vi "ABR3-Init Freq.vi"(0 "StimChans":T5[](xcontrol), 1 "Runtime":T28={"Ceiling"=0.0, "Threshold"=0.0, "Crossed?"=FALSE, "Step"=0, "Stop"=0, "Avgs"=0, "Level"=0.0, "AI Npts"=0, "Doubled?"=FALSE, "Gain"=0.0, "NWindowPts"=0, "dt"=0.0, "Cal"=path "", "Freq"=0.0, "AO Channels"=[], "AltPol"=FALSE, "AO Npts"=0, "AO Fs"=0.0, "Start"=0, "Stop max"=0, "Ear"=enum."Right", "Waveform"=enum."TONE PIP", "RepRate"=0.0, "CAP or ABR"=1, "LMasker"=0.0, "SeqVar"=enum."Signal Level", "Reps/buffer"=0, "Avg Mode"=enum."Neural/CM", "Wav"=path "", "Order"=enum."Sequential", "Levels"=[], "ControlVal"=0.0, "innerIndex"=0, "indexStep"=0} {"CAP or ABR" items=["CAP", "ABR"]}, 2 "State (in)":T2, 7 "outerVal":cluster{"wavfile":path, "freq":dbl}, 11 "error in (no error)":errorcluster, 12 "Response":T32={"Gain"=10000, "Averages"=1, "Window (ms)"=512.0, "Thr Fast Steps"=8.5, "AI Fs"=0.0} {"Thr Fast Steps" format="%.2f"; "Window (ms)" format="%.2f"}, 13 "Controls":T1) -> (3 "Runtime out":T28={"Ceiling"=0.0, "Threshold"=0.0, "Crossed?"=FALSE, "Step"=0, "Stop"=0, "Avgs"=0, "Level"=0.0, "AI Npts"=0, "Doubled?"=FALSE, "Gain"=0.0, "NWindowPts"=0, "dt"=0.0, "Cal"=path "", "Freq"=0.0, "AO Channels"=[], "AltPol"=FALSE, "AO Npts"=0, "AO Fs"=0.0, "Start"=0, "Stop max"=0, "Ear"=enum."Right", "Waveform"=enum."TONE PIP", "RepRate"=0.0, "CAP or ABR"=1, "LMasker"=0.0, "SeqVar"=enum."Signal Level", "Reps/buffer"=0, "Avg Mode"=enum."Neural/CM", "Wav"=path "", "Order"=enum."Sequential", "Levels"=[], "ControlVal"=0.0, "innerIndex"=0, "indexStep"=0} {"CAP or ABR" items=["CAP", "ABR"]}, 4 "Stimulus (out)":T5[](xcontrol), 8 "Masker Level":T3, 10 "Ceiling":dbl, 15 "error out":errorcluster)   [LabVIEW 2020]
uses:
  TypeDefs/ABR3-Response.ctl
  epl-vi-lib/Signal Synthesis VIs/Controls/Multichannel (Full)/Multichannel (Full).xctl
  TypeDefs/ABR3-Runtime Data.ctl
  epl-vi-lib/Utility VIs/Type Defs/Left-Right ring.ctl
  TypeDefs/ABR-Waveform Enum.ctl
  TypeDefs/ABR3-Seq Var Enum.ctl
  epl-vi-lib/Signal Synthesis VIs/Controls/Level XCtl/Level Data.ctl
  epl-vi-lib/Signal Synthesis VIs/Controls/Level XCtl/Level Units.ctl
  CFTS Main Panel SubVIs/CFTS-Experiment State.ctl
  TypeDefs/ABR3-Controls.ctl
  epl-vi-lib/Signal Synthesis VIs/Controls/Waveform XCtl/Waveform Enum.ctl
  epl-vi-lib/Signal Synthesis VIs/Top Level VIs/Stimulus-Initialize (full).vi
  epl-vi-lib/Signal Synthesis VIs/Controls/Level XCtl/Level XCtl.xctl
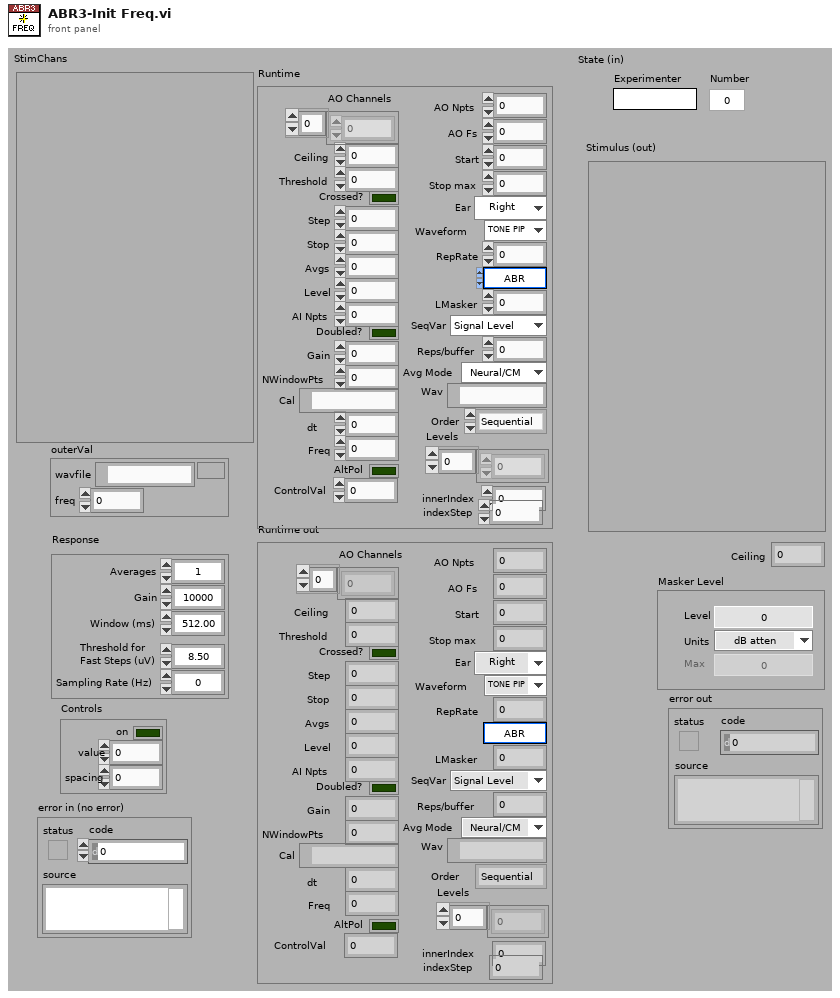
[diagram p1: front panel]
types:
  T1 = typedef "ABR3-Controls.ctl" = cluster{"on":bool, "value":dbl, "spacing":i32}
  T2 = typedef "CFTS-Experiment State.ctl" = cluster{"Experimenter":string, "Number":u32, "Right":string, "Left":string, "Data Folder":path, "State File":path, "Version Info":string, "End Exposure Time":dbl, "Exposure Duration":string, "Run #":cluster{"CAP":i16, "ABR":i16, "DP":i16, "VsEP":i16, "MeasSeq":i16, "SubSeq":i16, "SFOAE":i16}}
  T3 = typedef "Level XCtl.xctl/Level Data.ctl" = cluster{"Level":dbl, "Units":T4, "Max":dbl, "Multiplier":dbl, "Cal File":path, "Cal":cluster{"Freq (Hz)":dbl[], "Mag (dB SPL)":dbl[], "Phase (deg)":dbl[]}}
  T4 = typedef "Level Units.ctl" = enum16{"dB atten", "dB SPL", "dB re 1 Vrms", "dB V/Hz½", "mW", "dB HL", "Volts", "dB mW"}
  T5 = typedef "Stimulus Channel (Full).xctl/Full Stimulus Channel Data.ctl" = cluster{"Waveform":T6, "Filter":T23, "Burst":T25, "Level":T3, "Name":string, "Advanced":T26, "SAM":T27}
  T6 = typedef "Waveform XCtl.xctl/Waveform Data.ctl" = cluster{"Type":T7, "Tone":T8, "Pulse Train":T9, "Noise":T12, "File":T13, "FMSweep":T14, "Chirp Train":T15, "Complex Tone":cluster{"Params":T17, "Data":T19}, "Moving Ripple":T20}
  T7 = typedef "Waveform Enum.ctl" = enum16{"OFF", "Tone", "Noise", "Pulse Train", "File", "FM Sweep", "Chirp Train", "Complex Tone", "FM Tone", "Moving Ripple"}
  T8 = typedef "Tone Params.ctl" = cluster{"Frequency (kHz)":dbl, "Last Freq":dbl, "Last Phase":dbl}
  T9 = typedef "Pulse Train Params.ctl" = cluster{"Pulse width (us)":dbl, "Pulse rate (Hz)":dbl, "Gap (ms)":dbl, "Polarity":T10, "PT State":T11, "Asynch":bool}
  T10 = typedef "Pulse Polarity.ctl" = enum16{"POS", "NEG", "POS-NEG", "NEG-POS"}
  T11 = typedef "PT-Continuous State.ctl" = cluster{"Template":dbl[], "Nperiod":i32, "Index":i32, "Pulse Rate (Hz)":dbl, "Phase (cycles)":dbl, "Noff":i32}
  T12 = typedef "Noise Params.ctl" = cluster{"InvFilt":bool, "Noise":dbl[], "CurPt":i32, "Aweight":bool, "Seed":i32, "afile":path}
  T13 = typedef "StimFile-Params.ctl" = cluster{"Filename":path, "Signal":dbl[], "Channel":i32, "stream":bool, "offset":i32, "nreps":i32, "loops":i32, "Randomize":bool, "order":i32[], "Seed":i32, "Tokens":i32}
  T14 = typedef "FM Sweep Params.ctl" = cluster{"Rate (oct/s)":dbl, "Fmin (Hz)":dbl, "Fmax (Hz)":dbl, "Ramp (ms)":dbl, "Linear":bool}
  T15 = typedef "Chirp Train.ctl" = cluster{"Params":T16, "Data":cluster{"WF":dbl[]}}
  T16 = typedef "Chirp Train Params.ctl" = cluster{"Fmin (kHz)":dbl, "Fmax (kHz)":dbl, "Compensate":bool, "Duration (ms)":dbl}
  T17 = typedef "CT-Params.ctl" = cluster{"F0 (Hz)":dbl, "Band":cluster{"Flow (Hz)":dbl, "Fhigh (Hz)":dbl}, "Phase":T18, "Min F0 (Hz)":dbl, "Max F0 (Hz)":dbl, "ContinRandPhase":bool, "Max peak factor":dbl, "Max mod depth":dbl, "MinHarmNum":i32, "MaxHarmNum":i32, "Level Mode":enum16{"per component", "overall rms"}, "% jitter":dbl}
  T18 = typedef "CT-Phase Enum.ctl" = enum16{"Cosine", "Random", "Alternating"}
  T19 = typedef "CT-Runtime Data.ctl" = cluster{"Ncomp":i32, "MinHarm":i32, "Phase":dbl[], "Amplitude":dbl[], "Npts/frame":i32, "Last F0":dbl, "Fmin":dbl, "Fmax":dbl, "Lslope":dbl, "randphase":bool, "overall rms":bool, "fmult":dbl[], "jittered":bool}
  T20 = typedef "Moving Ripple.ctl" = cluster{"Params":T21, "Data":T22}
  T21 = typedef "Moving Ripple.Params.ctl" = cluster{"Fmin":dbl, "Fmax":dbl, "Density":dbl, "Velocity":dbl, "Depth":dbl, "Phase":dbl, "Comp/oct":i32}
  T22 = typedef "Moving Ripple.Data.ctl" = cluster{"Freq":dbl[], "A":dbl[], "phase":dbl[], "Phase":dbl}
  T23 = typedef "Advanced Filter XCtl.xctl/Filter Data.ctl" = cluster{"Type":enum16{"Lowpass", "Highpass", "Bandpass", "Bandstop", "OFF"}, "CF (kHz)":dbl, "BW (kHz)":dbl, "Cascade":bool, "Quadrature":bool, "Scale Factor":dbl, "Stages":cluster{"IIR Filter":cluster{"filter structure":enum32{"IIR 2nd Order", "IIR 4th Order"}, "Reverse Coefficients":dbl[], "Forward Coefficients":dbl[]}, "State":dbl[]}[], "Class":enum16{"Elliptic", "Butterworth"}, "Order":i32, "BWUnits":T24}
  T24 = typedef "Filter-Bandwidth Units.ctl" = enum16{"Linear", "Octaves", "Min-Max"}
  T25 = typedef "Burst Control.xctl/Burst Data.ctl" = cluster{"Active":bool, "Delay (ms)":dbl, "Duration (ms)":dbl, "Ramp (ms)":dbl, "Rate (Hz)":dbl, "Trepeat (ms)":dbl, "Repeat":bool}
  T26 = typedef "Advanced Stimulus Options.xctl/Advanced Stimulus Options.ctl" = cluster{"Rep Mask":string, "AltPol":bool, "Var":string, "Expr":string, "Persist":bool}
  T27 = typedef "SAM Params.ctl" = cluster{"Active":bool, "Frequency (Hz)":dbl, "Depth":dbl, "Init Phase (cycles)":dbl, "phase (degrees)":dbl, "Asynch":bool}
  T28 = typedef "ABR3-Runtime Data.ctl" = cluster{"Ceiling":dbl, "Threshold":dbl, "Crossed?":bool, "Step":i32, "Stop":i32, "Avgs":i32, "Level":dbl, "AI Npts":i32, "Doubled?":bool, "Gain":dbl, "NWindowPts":i32, "dt":dbl, "Cal":path, "Freq":dbl, "AO Channels":i32[], "AltPol":bool, "AO Npts":i32, "AO Fs":dbl, "Start":i32, "Stop max":i32, "Ear":T29, "Waveform":T30, "RepRate":dbl, "CAP or ABR":u16, "LMasker":dbl, "SeqVar":T31, "Reps/buffer":i32, "Avg Mode":enum16{"Neural/CM", "ANOW"}, "Wav":path, "Order":enum16{"Sequential", "Random"}, "Levels":dbl[], "ControlVal":dbl, "innerIndex":i32, "indexStep":i32}
  T29 = typedef "Left-Right ring.ctl" = enum16{"Right", "Left"}
  T30 = typedef "ABR-Waveform Enum.ctl" = enum16{"TONE PIP", "CLICK", "FILE", "CHIRP", "NOISE", "VERHULST"}
  T31 = typedef "ABR3-Seq Var Enum.ctl" = enum16{"Signal Level", "Masker Level"}
  T32 = typedef "ABR3-Response.ctl" = cluster{"Gain":i32, "Averages":i32, "Window (ms)":sgl, "Thr Fast Steps":sgl, "AI Fs":dbl}
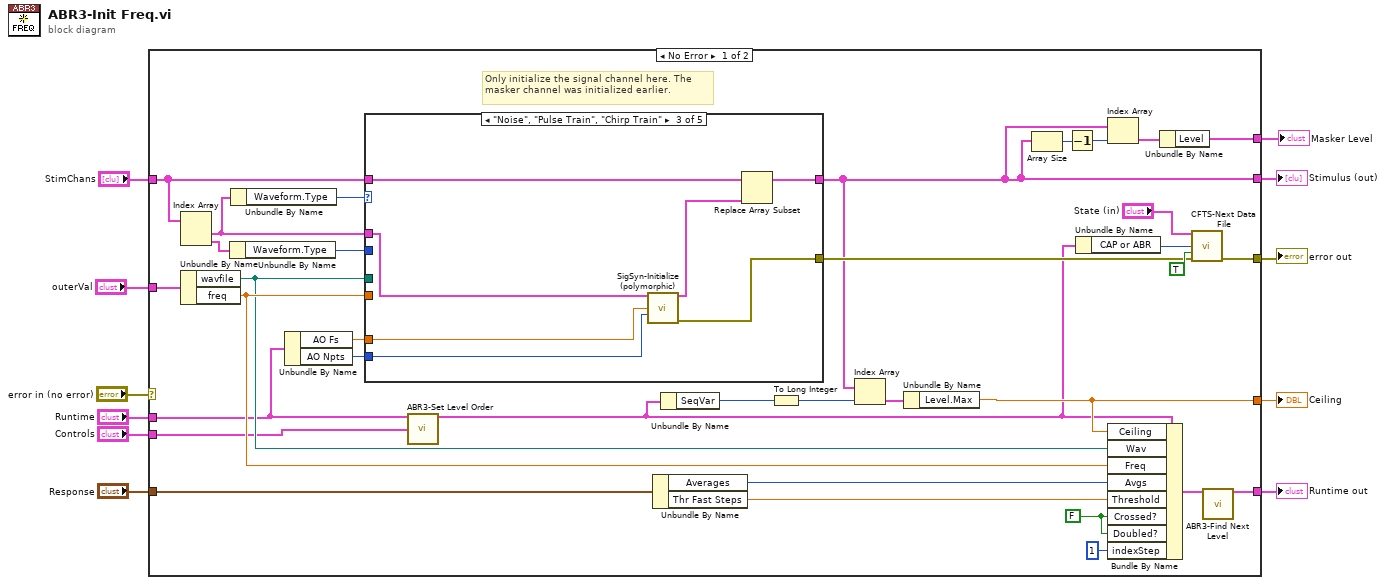
[diagram p0: block diagram]
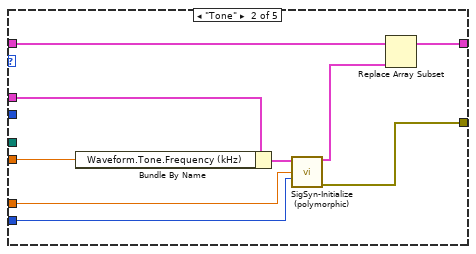
[diagram p3: hidden frame]
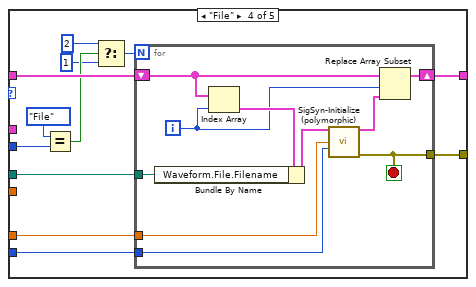
[diagram p4: hidden frame]
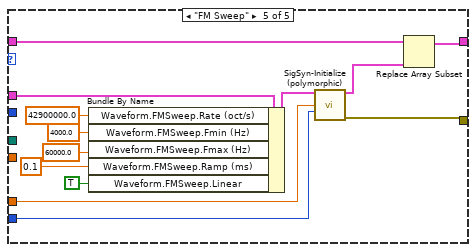
[diagram p5: hidden frame]
diagram:
  n1 = case shown="No Error" "error in (no error)" {
    selector: "error in (no error)" -> [_ w98]
    tunnel: "Response" -> [w45 _]
    tunnel: [w13 _] -> w10
    tunnel: [w40 _] -> w9
    tunnel: [w34 w98] -> w8
    tunnel: [w30 _] -> w7
    tunnel: "Runtime" -> [w17 _]
    tunnel: [w25 _] -> w5
    tunnel: "StimChans" -> [w29 _]
    tunnel: "outerVal" -> [w20 _]
    tunnel: "Controls" -> [w16 _]
    frame No Error {
      w44 = FALSE ("Crossed?")
      # "Only initialize the signal channel here. The masker channel was initialized earlier."
      n2 = Index Array(array=w29) -> (element #1=w32:T5, element #2=w28:T5)  [unwired: 2 in]
      n3 = Unbundle By Name(w20) -> ("wavfile"=w18:path, "freq"=w19:dbl)
      n4 = Unbundle By Name(w28) -> ("Waveform.Type"=w27:T7)
      n5 = Unbundle By Name(w32) -> ("Waveform.Type"=w31:T7)
      n6 = Unbundle By Name(w17) -> ("AO Fs"=w22:dbl, "AO Npts"=w21:i32)
      n7 = case shown="\"Noise\", \"Pulse Train\", \"Chirp Train\"" w31 {
        tunnel: w19 -> [_ w55 _ _ _]
        tunnel: w32 -> [_ w54 w62 _ w97]
        tunnel: w18 -> [_ _ _ w74 _]
        tunnel: w29 -> [w46 w53 w61 w73 w91]
        tunnel: [w46 w52 w60 w70 w90] -> w25
        tunnel: w27 -> [_ _ _ w72 _]
        tunnel: [_ w49 w58 w69 w87] -> w26
        tunnel: w22 -> [_ w48 w57 w64 w86]
        tunnel: w21 -> [_ w47 w56 w63 w85]
        frame "OFF", Default {
        }
        frame "Tone" {
          n8 = Bundle By Name(cluster=w54, "Waveform.Tone.Frequency (kHz)"=w55) -> (w51:T5)
          n9 = call-poly "SigSyn-Initialize (polymorphic).vi"("Stimulus Channel"=w51, "Sampling rate (Hz)"=w48, "Npts"=w47) -> ("Stimulus Channel out"=w50:T5, "error out"=w49:errorcluster)  [unwired: 10 in, 1 out]
          n10 = Replace Array Subset(array=w53, new element=w50) -> (w52:T5[])  [unwired: 1 in]
        }
        frame "Noise", "Pulse Train", "Chirp Train" {
          n11 = call-poly "SigSyn-Initialize (polymorphic).vi"("Stimulus Channel"=w62, "Sampling rate (Hz)"=w57, "Npts"=w56) -> ("Stimulus Channel out"=w59:T5, "error out"=w58:errorcluster)  [unwired: 10 in, 1 out]
          n12 = Replace Array Subset(array=w61, new element=w59) -> (w60:T5[])  [unwired: 1 in]
        }
        frame "File" {
          n13 = Equal?(x=Waveform_Enum."File" ("y"), y=w72) -> (x = y?=w67:bool)
          n14 = Select(t=2, s=w67, f=1) -> (s? t:f=w68:i32)
          n15 = for {
            N: w68 -> [_]
            tunnel: w74 -> [w84]
            shift-right: [w82] -> w70
            shift-left: w73 -> [w80]
            tunnel: [w78] -> w69
            tunnel: w64 -> [w76]
            tunnel: w63 -> [w75]
            i -> [w77]
            stop <- w78 stop-if-true
            n16 = Index Array(array=w80, index=w77) -> (element=w79:T5)
            n17 = Bundle By Name(cluster=w79, "Waveform.File.Filename"=w84) -> (w83:T5)
            n18 = call-poly "SigSyn-Initialize (polymorphic).vi"("Stimulus Channel"=w83, "Sampling rate (Hz)"=w76, "Npts"=w75) -> ("Stimulus Channel out"=w81:T5, "error out"=w78:errorcluster)  [unwired: 10 in, 1 out]
            n19 = Replace Array Subset(array=w80, new element=w81, index=w77) -> (w82:T5[])
          }
        }
        frame "FM Sweep" {
          n20 = Bundle By Name(cluster=w97, "Waveform.FMSweep.Rate (oct/s)"=42900000.0, "Waveform.FMSweep.Fmin (Hz)"=4000.0, "Waveform.FMSweep.Fmax (Hz)"=60000.0, "Waveform.FMSweep.Ramp (ms)"=0.1, "Waveform.FMSweep.Linear"=TRUE) -> (w89:T5)
          n21 = call-poly "SigSyn-Initialize (polymorphic).vi"("Stimulus Channel"=w89, "Sampling rate (Hz)"=w86, "Npts"=w85) -> ("Stimulus Channel out"=w88:T5, "error out"=w87:errorcluster)  [unwired: 10 in, 1 out]
          n22 = Replace Array Subset(array=w91, new element=w88) -> (w90:T5[])  [unwired: 1 in]
        }
      }
      n23 = call "ABR3-Set Level Order.vi"("Runtime In"=w17, "Controls"=w16) -> ("Runtime Out"=w15:T28)  [unwired: 13 in]
      n24 = Unbundle By Name(w45) -> ("Averages"=w43:i32, "Thr Fast Steps"=w42:sgl)
      n25 = Unbundle By Name(w15) -> ("SeqVar"=w39:T31)
      n26 = To Long Integer(number=w39) -> (32bit integer=w38:i32)
      n27 = Index Array(array=w25, index=w38) -> (element=w37:T5)
      n28 = Unbundle By Name(w37) -> ("Level.Max"=w30:dbl)
      n29 = Array Size(array=w25) -> (size(s)=w24:i32)
      n30 = Decrement(x=w24) -> (x-1=w23:i32)
      n31 = Unbundle By Name(w15) -> ("CAP or ABR"=w33:u16)
      n32 = Index Array(array=w25, index=w23) -> (element=w41:T5)
      n33 = Bundle By Name(cluster=w15, "Ceiling"=w30, "Wav"=w18, "Freq"=w19, "Avgs"=w43, "Threshold"=w42, "Crossed?"=w44, "Doubled?"=w44, "indexStep"=1) -> (w14:T28)
      n34 = Unbundle By Name(w41) -> ("Level"=w40:T3)
      n35 = call "CFTS-Next Data File.vi"("Expt State"="State (in)", "Data Type"=w33, "Test only"=TRUE, "error in (no error)"=w26) -> ("error out"=w34:errorcluster)  [unwired: 7 in, 4 out]
      n36 = call "ABR3-Find Next Level.vi"("Runtime"=w14) -> ("Runtime out"=w13:T28)  [unwired: 12 in, 2 out]
    }
    frame Error {
    }
  }
  "error out" <- w8
  "Ceiling" <- w7
  "Runtime out" <- w10
  "Stimulus (out)" <- w5
  "Masker Level" <- w9
